vi "test Add EST CD Returns Successfully.vi"(8 "error in (no error)":errorcluster, 11 "TestCase in":refnum<class "Scripting API Test Case.lvclass">) -> (0 "error out":errorcluster, 3 "TestCase out":refnum<class "Scripting API Test Case.lvclass">)   [LabVIEW 2015, in "Scripting API Test Case.lvclass"]
uses:
  Scripting API Test Case.lvclass
  SysDef API/Engine Simulation Toolkit Custom Device Settings.ctl
  <vilib>/NI Veristand/Custom Device API/Custom Device Timed Loop Priority.ctl
  NationalInstruments.VeriStand.SystemDefinitionAPI
  <userlib>/_OpenG.lib/file/file.llb/Append Path to Root if Relative - Scalar__ogtk.vi
  <vilib>/addons/_JKI Toolkits/VI Tester/TestCase.llb/TestCase.lvclass
  SysDef API/Engine Simulation Toolkit SysDef API.lvlib
  <vilib>/NI Veristand/Custom Device API/Custom Device API.lvlib
  niveristand-custom-device-testing-tools/VeriStandTestUtilities/VeriStandTestUtilities.lvlib
panel:
  out "string":string
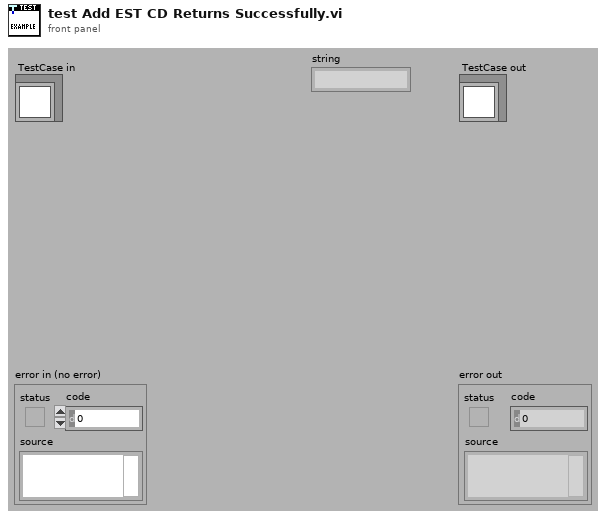
[diagram p1: front panel]
types:
  T1 = typedef "Engine Simulation Toolkit SysDef API.lvlib/Engine Simulation Toolkit Custom Device Settings.ctl" = cluster{"Name":string, "Execution priority":T2, "Rate decimation":i32, "CPU":i32, "Device address":string, "Bitfile path":path, "APUs":string[]}
  T2 = typedef "Custom Device API.lvlib/Custom Device Timed Loop Priority.ctl" = enum32{"Low", "Medium", "High"}
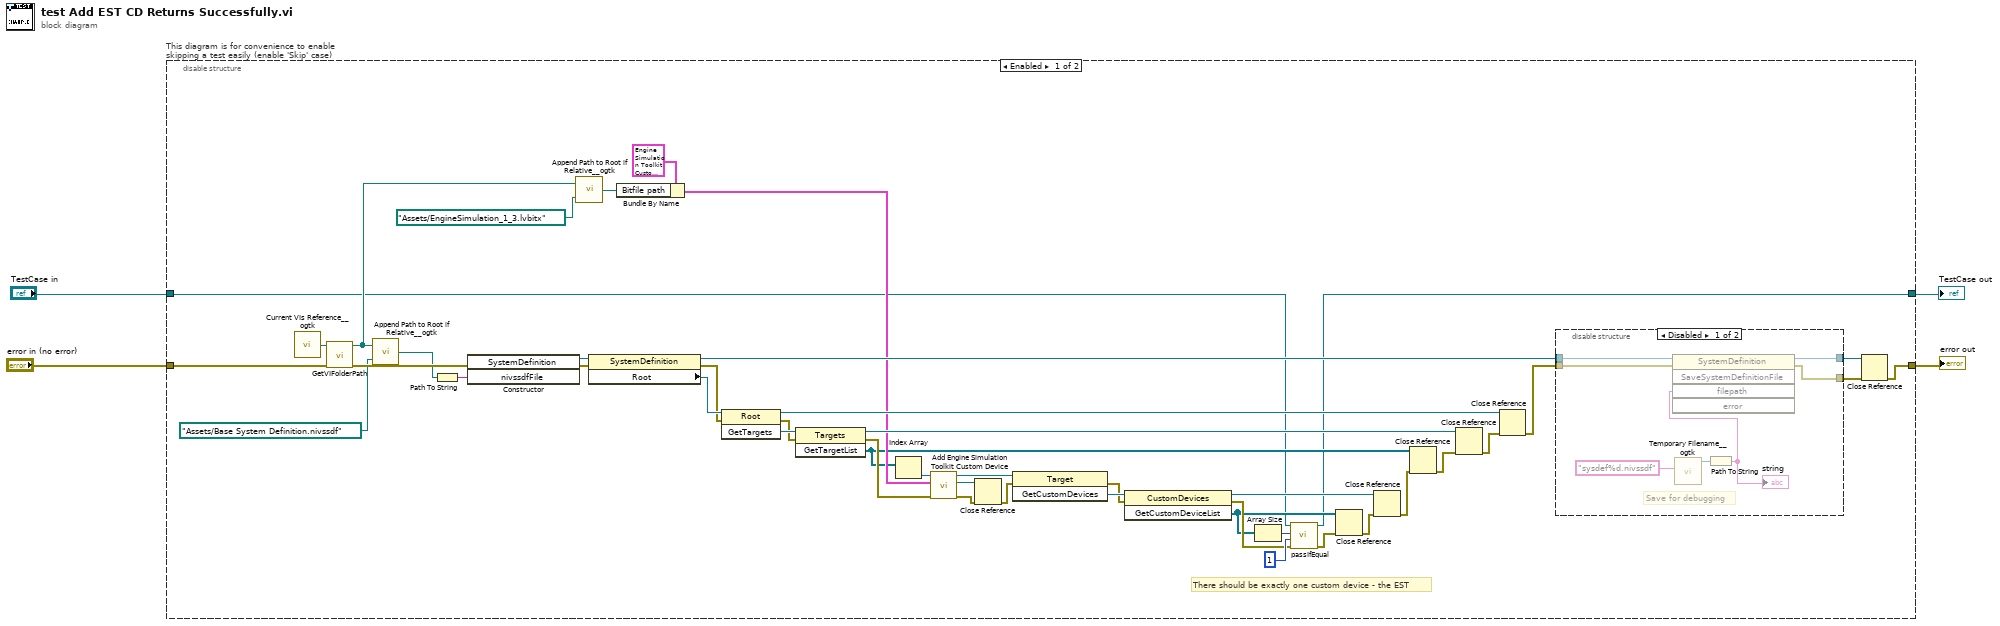
[diagram p0: block diagram]
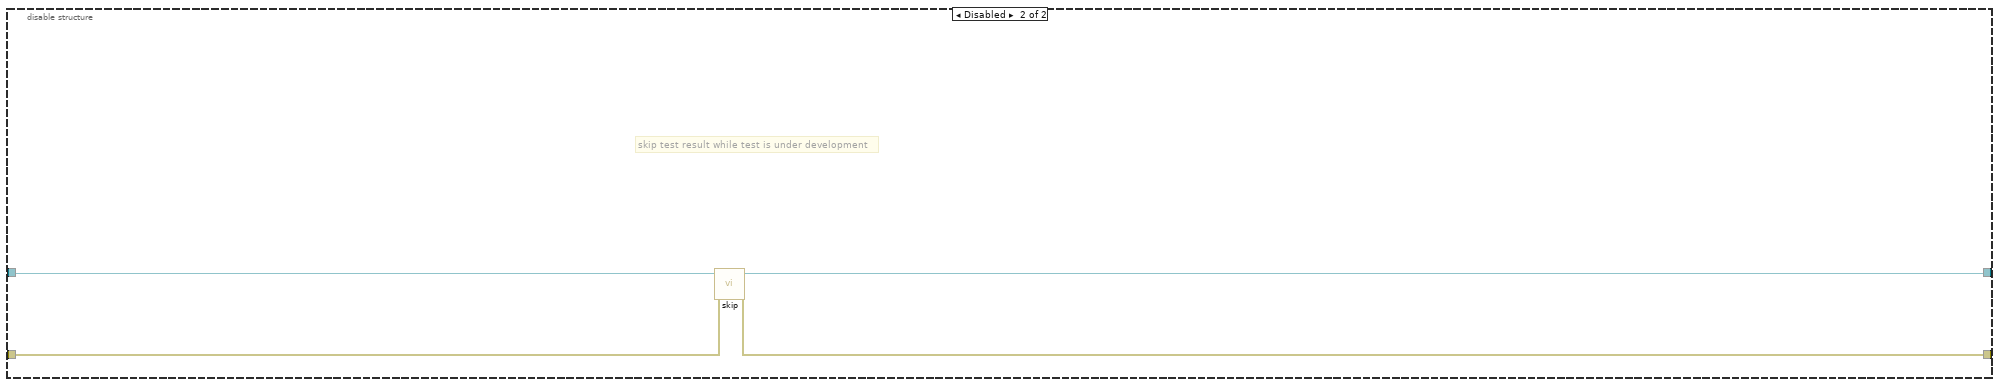
[diagram p3: hidden frame]
diagram:
  n1 = disable-structure "This diagram is for convenience to enable skipping a test easily (enable 'Skip' case)" shown="Enabled" {
    disable-tunnel: "TestCase in" -> [w6 w62]
    disable-tunnel: [w5 w60] -> w1
    disable-tunnel: [w41 w61] -> w3
    disable-tunnel: "error in (no error)" -> [w27 w59]
    frame Enabled {
      # "There should be exactly one custom device - the EST"
      n2 = call <userlib>:"Current VIs Reference__ogtk.vi"() -> ("Current VI's reference"=w28:refnum<vi>)  [unwired: 5 in]
      n3 = call "GetVIFolderPath.vi"("error in (no error)"=w27, "VI Reference in"=w28) -> ("error out"=w26:errorcluster, "VI Folder Path out"=w23:path)  [unwired: 8 in]
      n4 = call-poly <userlib>:"Append Path to Root if Relative__ogtk.vi"("Absolute or Relative Path"=path "Assets/Base System Definition.nivssdf", "Root Path"=w23) -> ("Absolute or Appended Path"=w24:path)
      n5 = Path To String(path=w24) -> (string=w29:string)
      n6 = constructor class="SystemDefinition"(error in=w26, "nivssdfFile"=w29) -> (reference out=w49:refnum<k24>, error out=w48:errorcluster)  [unwired: 2 in, 2 out]
      n7 = call-poly <userlib>:"Append Path to Root if Relative__ogtk.vi"("Absolute or Relative Path"=path "Assets/EngineSimulation_1_3.lvbitx", "Root Path"=w23) -> ("Absolute or Appended Path"=w30:path)
      n8 = property class="SystemDefinition"(reference=w49, error in=w48) -> (reference out=w42:refnum<k24>, error out=w44:errorcluster, "Root"=w47:refnum<k24>)
      n9 = Bundle By Name(cluster=T1 {"Name"="Engine Simulation Toolkit", "Execution priority"=enum."Medium", "Rate decimation"=1, "CPU"=-2, "Device address"="RIO 0", "Bitfile path"=path "", "APUs"=[]} ("Engine Simulation Toolkit Custom Device Settings"), "Bitfile path"=w30) -> (w32:T1)
      n10 = invoke class="Root" method="GetTargets"(reference=w47, error in=w44) -> (reference out=w37:refnum<k24>, error out=w45:errorcluster, "GetTargets"=w46:refnum<k24>)  [unwired: 1 in]
      n11 = invoke class="Targets" method="GetTargetList"(reference=w46, error in=w45) -> (reference out=w36:refnum<k24>, error out=w33:errorcluster, "GetTargetList"=w10:refnum<k24>[])  [unwired: 1 in]
      n12 = Index Array(array=w10) -> (element=w21:refnum<k24>)  [unwired: 1 in]
      n13 = call "Add Engine Simulation Toolkit Custom Device.vi"("error in (no error)"=w33, "Engine Simulation Toolkit Custom Device Settings"=w32, "Target in"=w21) -> ("error out"=w20:errorcluster, "EST Custom Device"=w22:refnum<k24>, "Target out"=w19:refnum<k24>)  [unwired: 6 in]
      n14 = Close Reference(reference=w22, error in (no error)=w20) -> (error out=w18:errorcluster)
      n15 = invoke class="Target" method="GetCustomDevices"(reference=w19, error in=w18) -> (error out=w16:errorcluster, "GetCustomDevices"=w17:refnum<k24>)  [unwired: 1 in, 1 out]
      n16 = invoke class="CustomDevices" method="GetCustomDeviceList"(reference=w17, error in=w16) -> (reference out=w7:refnum<k24>, error out=w12:errorcluster, "GetCustomDeviceList"=w11:refnum<k24>[])  [unwired: 1 in]
      n17 = Array Size(array=w11) -> (size(s)=w15:i32)
      n18 = call-dynamic "passIfEqual.vi"("error in (no error)"=w12, "y"=1 ("size(s)"), "x"=w15, "TestCase in"=w6) -> ("error out"=w13:errorcluster, "TestCase out"=w5:refnum<class "Scripting API Test Case.lvclass">)  [unwired: 6 in]
      n19 = Close Reference(reference=w11, error in (no error)=w13) -> (error out=w9:errorcluster)
      n20 = Close Reference(reference=w7, error in (no error)=w9) -> (error out=w8:errorcluster)
      n21 = Close Reference(reference=w10, error in (no error)=w8) -> (error out=w34:errorcluster)
      n22 = Close Reference(reference=w36, error in (no error)=w34) -> (error out=w35:errorcluster)
      n23 = Close Reference(reference=w37, error in (no error)=w35) -> (error out=w38:errorcluster)
      n24 = disable-structure shown="Disabled" {
        disable-tunnel: w42 -> [w56 w57]
        disable-tunnel: [w55 w58] -> w40
        disable-tunnel: [w54 w57] -> w39
        disable-tunnel: w38 -> [w53 w58]
        frame Disabled {
          # "Save for debugging"
          n25 = call <userlib>:"Temporary Filename__ogtk.vi"("pattern (lvtemp%d.tmp)"="sysdef%d.nivssdf") -> ("file in tmp dir"=w51:path)  [unwired: 5 in, 1 out]
          n26 = Path To String(path=w51) -> (string=w50:string)
          "string" <- w50
          n27 = invoke class="SystemDefinition" method="SaveSystemDefinitionFile"(reference=w56, error in=w53, "filepath"=w50) -> (reference out=w54:refnum<k24>, error out=w55:errorcluster)  [unwired: 2 in, 3 out]
        }
        frame Enabled {
        }
      }
      n28 = Close Reference(reference=w39, error in (no error)=w40) -> (error out=w41:errorcluster)
    }
    frame Disabled {
      # "skip test result while test is under development"
      n29 = call <vilib>:"skip.vi"("error in (no error)"=w59, "TestCase in"=w62) -> ("error out"=w61:errorcluster, "TestCase out"=w60:refnum<class "Scripting API Test Case.lvclass">)  [unwired: 8 in]
    }
  }
  "error out" <- w3
  "TestCase out" <- w1
